vi "Representation Ring to Enum.vi"(11 "Representation Ring":T1) -> (3 "Representation Enum":T2)   [LabVIEW 2018, in "Numeric Data Type.lvclass"]
uses:
  Numeric Data Type.lvclass
  Representation Enum.ctl
  Representation Ring.ctl
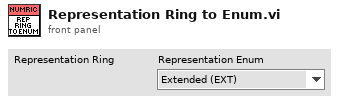
[diagram p1: front panel]
types:
  T1 = typedef "Numeric Data Type.lvclass/Representation Ring.ctl" = u16
  T2 = typedef "Numeric Data Type.lvclass/Representation Enum.ctl" = enum16{"Extended (EXT)", "Double (DBL)", "Single (SGL)", "Fixed-Point (FXP)", "Quad Integer (I64)", "Long Integer (I32)", "Word Integer (I16)", "Byte Integer (I8)", "Unsigned Quad (U64)", "Unsigned Long (U32)", "Unsigned Word (U16)", "Unsigned Byte (U8)", "Complex Extended (CXT)", "Complex Double (CDB)", "Complex Single (CSG)"}
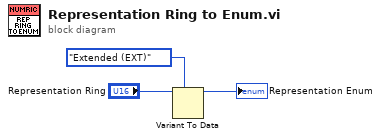
[diagram p0: block diagram]
diagram:
  n1 = Variant To Data(type=Representation_Enum."Extended (EXT)" ("Representation Enum"), Variant="Representation Ring") -> (data=→"Representation Enum":T2)  [unwired: 1 in, 1 out]
